vi "Acquire and logging - Copy.vi"() -> ()   [LabVIEW 2016]
uses:
  <vilib>/LabVIEW Interface for Arduino/LabVIEW Interface for Arduino.lvlib
panel:
  in  "Analog Input Pin":u8
  in  "Clear graph":bool
  out "pass time (min)":i16
  out "current time":timestamp
  out "start time":timestamp
  out "Waveform Chart 2":dbl[](graph)
  in  "Flush? (T)":bool=TRUE
  out "FFT":waveform(dbl)(graph)
  in  "Acquition Speed":u32
  in  "Filename":path=path "D:/do an nang cao/data.xlsx"
  in  "Gain":dbl=99.0 format="%#_13g"
  out "error out":errorcluster
  out "Waveform Chart":dbl[](graph)
  in  "VISA resource":refnum<visa-resource-name>
  in  "stop":bool
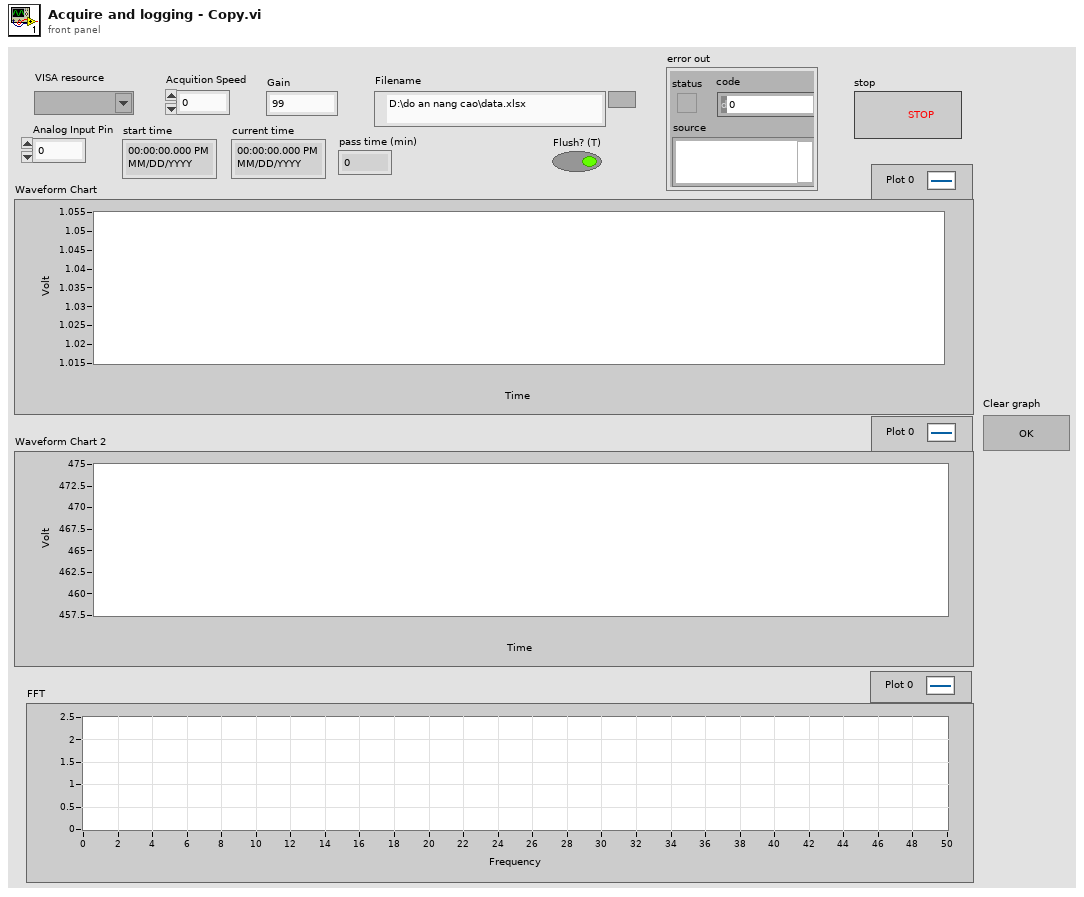
[diagram p1: front panel]
types:
  T1 = typedef "LabVIEW Interface for Arduino.lvlib/Arduino Resource.ctl" = cluster{"VISA resource":refnum<visa-resource-name>, "Board Type":T2, "Connection Type":enum8{"USB / Serial"}, "Bytes Per Packet (15)":u8}
  T2 = typedef "LabVIEW Interface for Arduino.lvlib/Board Type.ctl" = enum16{"Uno", "Dimuelanove w/Atmega 328", "Mega 2560"}
  T3 = typedef "LVDateTimeRec.ctl" = cluster{"fractional second":dbl, "second":i32, "minute":i32, "hour":i32, "day of month":i32, "month":i32, "year":i32, "day of week":i32, "day of year":i32, "DST":i32}
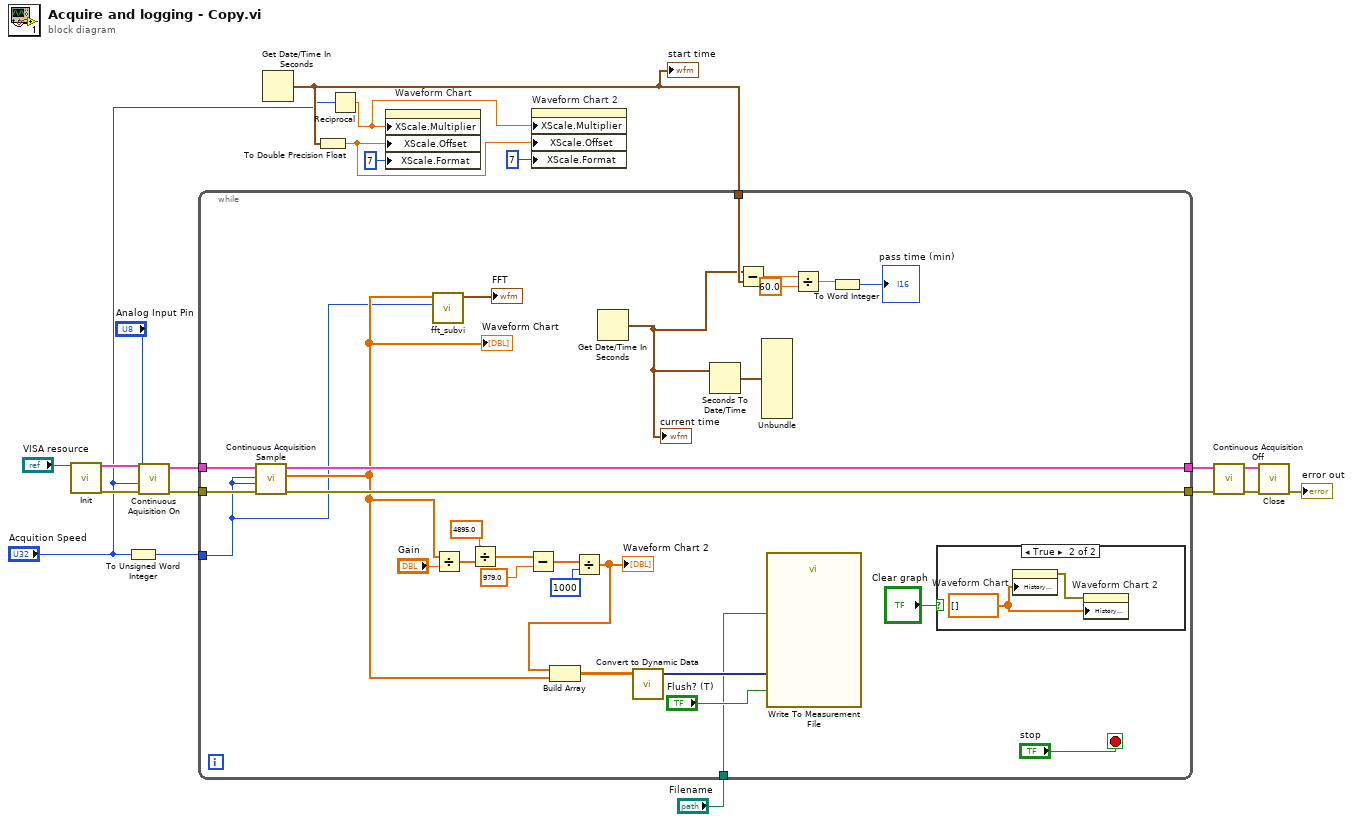
[diagram p0: block diagram]
diagram:
  n1 = call <vilib>:"Init.vi"("VISA resource"="VISA resource") -> ("Arduino Resource"=w19:T1, "error out"=w15:errorcluster)  [unwired: 17 in]
  n2 = To Unsigned Word Integer(number="Acquition Speed") -> (unsigned 16bit integer=w8:u16)
  n3 = call <vilib>:"Continuous Aquisition On.vi"("error in"=w15, "Acquition Speed"="Acquition Speed", "Analog Input Pin"="Analog Input Pin", "Arduino Resource"=w19) -> ("error out"=w14:errorcluster, "Arduino Resource"=w18:T1)  [unwired: 6 in]
  n4 = Get Date/Time In Seconds() -> (seconds since 1Jan1904=w2:timestamp)
  "start time" <- w2
  n5 = while {
    tunnel: w18 -> [w47]
    tunnel: [w46] -> w17
    tunnel: w14 -> [w45]
    tunnel: [w44] -> w13
    tunnel: w8 -> [w20]
    tunnel: "Filename" -> [w29]
    tunnel: w2 -> [w28]
    stop <- "stop" stop-if-true
    n6 = call <vilib>:"Continuous Acquisition Sample.vi"("Arduino Resource"=w47, "Samples to Read"=w20, "Sample Rate (HZ)"=w20, "error in (no error)"=w45) -> ("Arduino Resource"=w46:T1, "Data"=w34:dbl[], "error out"=w44:errorcluster)  [unwired: 4 in]
    "Waveform Chart" <- w34
    n7 = call "fft_subvi.vi"("Fs"=w20, "Array"=w34) -> ("Waveform Graph"=→"FFT":waveform(dbl))  [unwired: 9 in]
    n8 = Divide(x=w34, y="Gain") -> (x/y=w42:dbl[])
    n9 = Divide(x=4895.0, y=w42) -> (x/y=w40:dbl[])
    n10 = Subtract(x=w40, y=979.0 ("x")) -> (x-y=w38:dbl[])
    n11 = Divide(x=w38, y=1000) -> (x/y=w33:dbl[])
    "Waveform Chart 2" <- w33
    n12 = Build Array(w33, w34) -> (w36:dbl[][])
    n13 = Get Date/Time In Seconds() -> (seconds since 1Jan1904=w22:timestamp)
    "current time" <- w22
    n14 = call "Convert to Dynamic Data"("2D Array"=w36) -> ("Dynamic Data Type"=w30:dynamicdata)  [unwired: 3 in]
    n15 = Seconds To Date/Time(time stamp (now)=w22) -> (date time rec=w21:T3)  [unwired: 1 in]
    n16 = Subtract(x=w22, y=w28) -> (x-y=w27:dbl)
    n17 = Unbundle(w21) -> ()  [unwired: 10 out]
    n18 = call "Write To Measurement File"("Signals"=w30, "Flush? (T)"="Flush? (T)", "Filename"=w29) -> ()  [unwired: 14 in, 3 out]
    n19 = Divide(x=w27, y=60.0) -> (x/y=w25:dbl)
    n20 = To Word Integer(number=w25) -> (16bit integer=→"pass time (min)":i16)
    n21 = case shown="True" "Clear graph" {
      frame False {
      }
      frame True {
        w48 = dbl[] [] ("History Data")
        n22 = property on="Waveform Chart" class="WFChart (strict)"("History Data"=w48) -> (error out=w49:errorcluster)  [unwired: 2 in, 1 out]
        n23 = property on="Waveform Chart 2" class="WFChart (strict)"(error in=w49, "History Data"=w48) -> ()  [unwired: 1 in, 2 out]
      }
    }
  }
  n24 = To Double Precision Float(number=w2) -> (double precision float=w6:dbl)
  n25 = Reciprocal(x="Acquition Speed") -> (1/x=w3:dbl)
  n26 = property on="Waveform Chart" class="WFChart (strict)"("XScale.Multiplier"=w3, "XScale.Offset"=w6, "XScale.Format"=u8 7 ("X Scale.Display Format:Format")) -> ()  [unwired: 2 in, 2 out]
  n27 = property on="Waveform Chart 2" class="WFChart (strict)"("XScale.Multiplier"=w3, "XScale.Offset"=w6, "XScale.Format"=u8 7 ("X Scale.Display Format:Format")) -> ()  [unwired: 2 in, 2 out]
  n28 = call <vilib>:"Continuous Acquisition Off.vi"("error in"=w13, "Arduino Resource"=w17) -> ("error out"=w12:errorcluster, "Arduino Resource"=w16:T1)  [unwired: 8 in]
  n29 = call <vilib>:"Close.vi"("Arduino Resource"=w16, "error in"=w12) -> ("error out"=→"error out":errorcluster)  [unwired: 13 in]
